vi "Calculate.vi"(8 "error in":errorcluster caption="entrée d'erreur (pas d'erreur)", 9 "IndicePoint":i32, 11 "Experiment.lvclass In":refnum<class "Experiment.lvclass">) -> (0 "error out":errorcluster caption="sortie d'erreur", 2 "Données":dbl[](array[numeric]), 3 "Experiment.lvclass Out":refnum<class "Experiment.lvclass">)   [LabVIEW 2019, in "Experiment.lvclass"]
uses:
  Experiment.lvclass
  Experiment.lvclass/Experiment.ctl
  Calculations Class/Calculations.lvclass
  C:/Programmes Labview/LabscanV1A/DevicesClass/BaseDevice/BaseDevice.lvclass
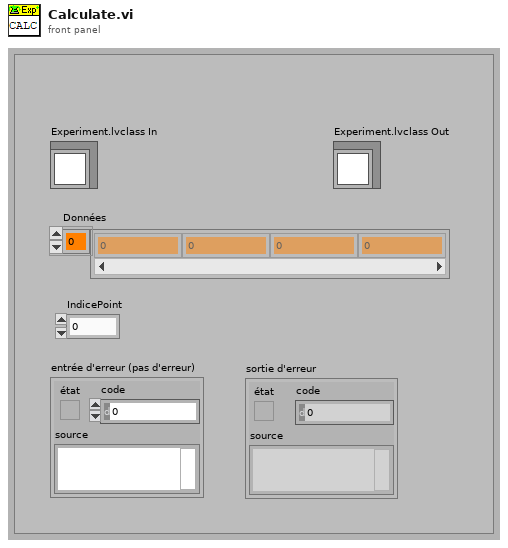
[diagram p1: front panel]
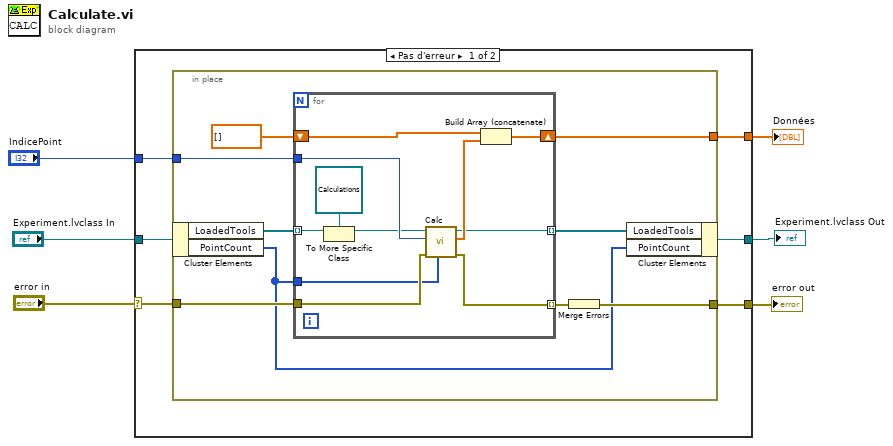
[diagram p0: block diagram]
diagram:
  n1 = case shown="Pas d'erreur" "error in" {
    selector: "error in" -> [w12 w34]
    tunnel: [w9 w34] -> w5
    tunnel: [w11 _] -> w4
    tunnel: "IndicePoint" -> [w10 _]
    tunnel: "Experiment.lvclass In" -> [w8 w33]
    tunnel: [w7 w33] -> w1
    frame No Error {
      n2 = in-place {
        in-place-border: w12 -> [w21]
        in-place-border: [w20] -> w11
        in-place-border: w10 -> [w15]
        in-place-border: [w18] -> w9
        n3 = in-place-cluster #1(w8) -> ("LoadedTools"=w17:refnum<class "BaseDevice.lvclass">[], "PointCount"=w13:i32[])
        n4 = for {
          tunnel: w21 -> [w29]
          tunnel: w15 -> [w26]
          shift-right: [w32] -> w20
          shift-left: dbl[] [] -> [w31]
          tunnel: w17 -> [w30] mode=indexing
          tunnel: [w27] -> w16 mode=indexing
          tunnel: [w25] -> w14 mode=indexing
          tunnel: w13 -> [w24]
          n5 = To More Specific Class(target class=refnum<class "Calculations.lvclass"> refnum ("Calculations.lvclass"), reference=w30) -> (specific class reference=w23:refnum<class "Calculations.lvclass">)  [unwired: 1 in, 1 out]
          n6 = call-dynamic "Calc.vi"("ScanTableSize"=w24, "error in (no error)"=w29, "AllPointIndex"=w26, "InstrClassIn"=w23) -> ("error out"=w25:errorcluster, "MeasDatOut"=w28:dbl[], "InstrClassOut"=w27:refnum<class "Calculations.lvclass">)  [unwired: 5 in]
          n7 = Build Array (concatenate)(w31, w28) -> (w32:dbl[])
        }
        n8 = Merge Errors(w14) -> (w18:errorcluster)
        n9 = in-place-cluster #1("LoadedTools"=w16, "PointCount"=w13) -> (w7:refnum<class "Experiment.lvclass">)
      }
    }
    frame Error {
    }
  }
  "error out" <- w5
  "Données" <- w4
  "Experiment.lvclass Out" <- w1
